vi "Test Process Retains State when Stopped from Branch.vi"(8 "error in (no error)":errorcluster, 11 "Process Test In":refnum<class "Process Dev Test.lvclass">) -> (0 "error out":errorcluster, 3 "Process Test Out":refnum<class "Process Dev Test.lvclass">)   [LabVIEW 2020, in "Process Dev Test.lvclass"]
uses:
  Process Dev Test.lvclass
  C:/Program Files (x86)/National Instruments/LabVIEW 2020/vi.lib/Astemes/LUnit/Test Case.lvclass
  source/Framework Test Suite/Mock Error Handler/Mock Error Handler.lvclass
  C:/Git/astemes-triarc-framework/source/Framework/Error Handler Interface/Error Handler Interface.lvclass
  source/Framework/Process/Process.lvclass/Process.ctl
  <vilib>/Astemes/LUnit/Test Case.lvclass/Test Case.ctl
  <vilib>/Astemes/LUnit/LUnit Assertion Result.lvclass/LUnit Assertion Result.ctl
  <vilib>/Astemes/LUnit/LUnit Test Case Result.lvclass/LUnit Test Case Result.ctl
  <vilib>/Astemes/LUnit/LUnit Method Result.lvclass/LUnit Method Result.ctl
  source/Framework/Process/Protected/Messaging/Enqueue Message.vi
  source/Framework/Process/Public/Lifecycle/Get Lifecycle State.vi
  source/Framework/Process/Private/SubVIs/Wait for finish.vi
  source/Framework/Process/Private/SubVIs/Set Lifecycle State.vi
  <vilib>/Astemes/LUnit/Set Assertion Type.vi
  <vilib>/Astemes/LUnit/Palette/Pass.vi
  <vilib>/Astemes/LUnit/Palette/Fail.vi
  source/Framework/Process/Private/SubVIs/Handle Debug Data.vi
  <vilib>/Utility/error.llb/Clear Errors.vi
  <vilib>/Astemes/LUnit/LUnit Write Assertion Type.vi
  <vilib>/Astemes/LUnit/Add test result.vi
  <vilib>/Astemes/LUnit/LUnit Write Passed.vi
  <vilib>/Astemes/LUnit/LUnit Write Message.vi
  <vilib>/Astemes/LUnit/LUnit Write Description.vi
  source/Framework/Logging/Log Debug.vi
  <vilib>/AdvancedString/1D String Array to Delimited String.vi
  <vilib>/Utility/High Resolution Relative Seconds.vi
  <vilib>/Astemes/LUnit/LUnit Record Assertion Result.vi
  <vilib>/Astemes/LUnit/LUnit Aggregate Assertion Results.vi
  <vilib>/Astemes/LUnit/Assertion Result/LUnit Read Status.vi
  <vilib>/Astemes/LUnit/LUnit Read Message.vi
  <vilib>/Astemes/LUnit/LUnit Read Description.vi
  <vilib>/Astemes/LUnit/Method Result/LUnit Merge Status.vi
  <vilib>/Astemes/LUnit/LUnit Concatenate result strings.vi
  <vilib>/Utility/error.llb/Error Cluster From Error Code.vi
  source/Framework/Process/Public/Read Name.vi
  <vilib>/Astemes/LUnit/LUnit Assertion Result.lvclass
  source/Framework/Process/Process.lvclass
  <vilib>/Astemes/LUnit/Test Case.lvclass
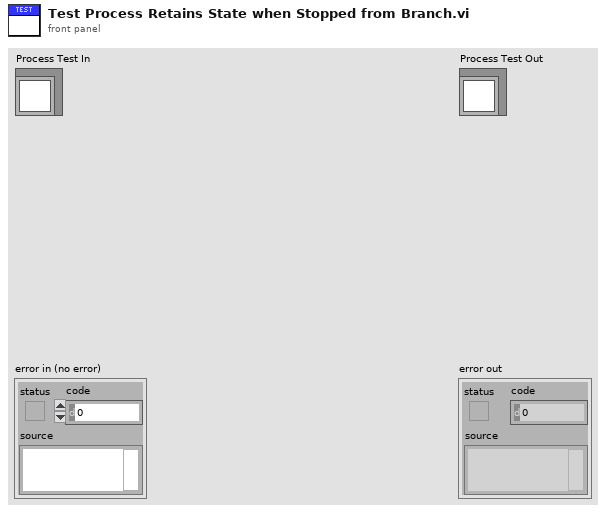
[diagram p1: front panel]
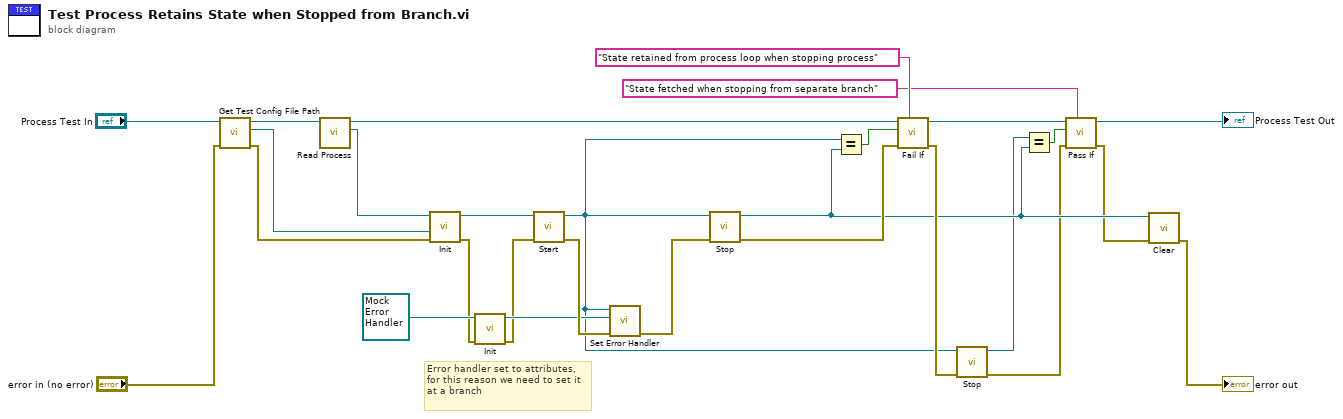
[diagram p0: block diagram]
diagram:
  # "Error handler set to attributes, for this reason we need to set it at a branch"
  n1 = call "Get Test Config File Path.vi"("error in (no error)"="error in (no error)", "Process Test In"="Process Test In") -> ("error out"=w24:errorcluster, "Test config path"=w27:path, "Process Test Out"=w28:refnum<class "Process Dev Test.lvclass">)  [unwired: 7 in]
  n2 = call "Read Process.vi"("Process Test in"=w28) -> ("Process.lvclass"=w25:refnum<class "Process.lvclass">, "Process Test out"=w26:refnum<class "Process Dev Test.lvclass">)  [unwired: 8 in, 1 out]
  n3 = call-dynamic "Init.vi"("error in (no error)"=w24, "Config File Path"=w27, "Process In"=w25) -> ("error out"=w13:errorcluster, "Process Out"=w17:refnum<class "Process.lvclass">)  [unwired: 7 in]
  n4 = call-dynamic "Init.vi"("error in (no error)"=w13, "Mock Error Handler In"=refnum<class "Mock Error Handler.lvclass"> refnum ("Mock Error Handler.lvclass")) -> ("error out"=w12:errorcluster, "Mock Error Handler Out"=w14:refnum<class "Mock Error Handler.lvclass">)  [unwired: 8 in]
  n5 = call "Start.vi"("error in (no error)"=w12, "Process In"=w17) -> ("error out"=w19:errorcluster, "Process Out"=w8:refnum<class "Process.lvclass">)  [unwired: 7 in, 1 out]
  n6 = call "Set Error Handler.vi"("error in (no error)"=w19, "Error Handler"=w14, "Process In"=w8) -> ("error out"=w18:errorcluster)  [unwired: 7 in, 1 out]
  n7 = call "Stop.vi"("error in (no error)"=w18, "Process In"=w8) -> ("error out"=w10:errorcluster, "Process Out"=w5:refnum<class "Process.lvclass">)  [unwired: 7 in, 1 out]
  n8 = Equal?(x=w8, y=w5) -> (x = y?=w15:bool)
  n9 = call <vilib>:"Fail If.vi"("Description"="State retained from process loop when stopping process", "error in (no error)"=w10, "Fail?"=w15, "LUnit Test Case In"=w26) -> ("error out"=w9:errorcluster, "LUnit Test Case Out"=w21:refnum<class "Process Dev Test.lvclass">)  [unwired: 6 in]
  n10 = call "Stop.vi"("error in (no error)"=w9, "Process In"=w8) -> ("error out"=w2:errorcluster, "Process Out"=w4:refnum<class "Process.lvclass">)  [unwired: 7 in, 1 out]
  n11 = Equal?(x=w4, y=w5) -> (x = y?=w3:bool)
  n12 = call <vilib>:"Pass If.vi"("Description"="State fetched when stopping from separate branch", "error in (no error)"=w2, "Pass?"=w3, "LUnit Test Case In"=w21) -> ("error out"=w1:errorcluster, "LUnit Test Case Out"=→"Process Test Out":refnum<class "Process Dev Test.lvclass">)  [unwired: 6 in]
  n13 = call-dynamic "Clear.vi"("error in (no error)"=w1, "Process In"=w5) -> ("error out"=→"error out":errorcluster)  [unwired: 9 in]
